vi "Write Control Panel Reference.vi"(8 "error in (no error)":errorcluster, 10 "Reference":refnum<vi>, 11 "Generic Controller in":refnum<class "Generic Plugin.lvclass">) -> (0 "error out":errorcluster, 3 "Generic Controller out":refnum<class "Generic Plugin.lvclass">)   [LabVIEW 2020, in "Generic Plugin.lvclass"]
uses:
  Generic Plugin.lvclass
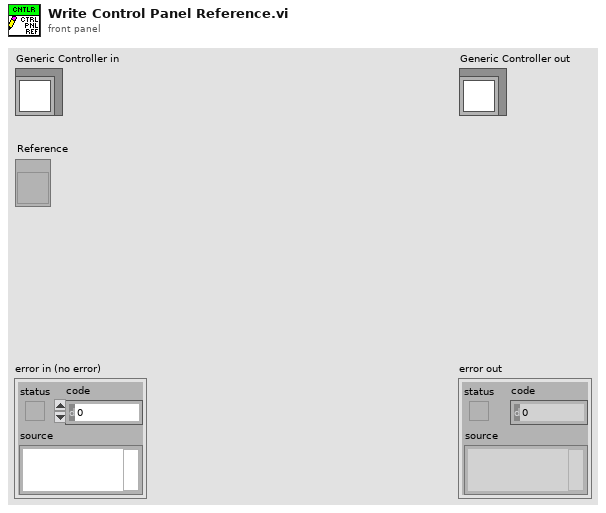
[diagram p1: front panel]
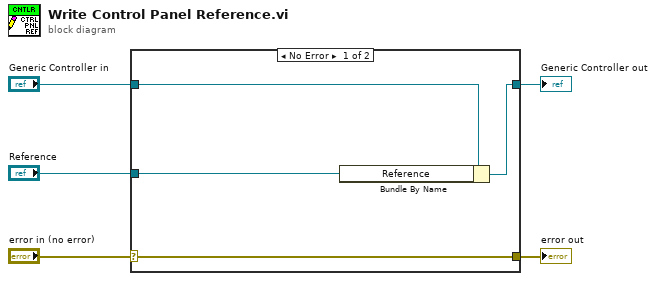
[diagram p0: block diagram]
diagram:
  n1 = case shown="No Error" "error in (no error)" {
    selector: "error in (no error)" -> [w9 w10]
    tunnel: [w9 w10] -> w4
    tunnel: [w7 w11] -> w2
    tunnel: "Generic Controller in" -> [w8 w11]
    tunnel: "Reference" -> [w6 _]
    frame No Error {
      n2 = Bundle By Name(cluster=w8, "Reference"=w6) -> (w7:refnum<class "Generic Plugin.lvclass">)
    }
    frame Error {
    }
  }
  "error out" <- w4
  "Generic Controller out" <- w2
